vi "Cryotel set mode.vi"() -> ()   [LabVIEW 2019]
panel:
  in  "PWOUT":dbl
  out "Step #":i32
  out "Command sent":string
  in  "milliseconds to wait":u32=1000
  out "read string array 2":string[](array[string])
  in  "Select command set":u16(ring) items=["Satus", "Constant power", "Target temperature", "Cooler OFF ", "Cooler ON", "Set power "]
  out "read string array":string[](array[string])
  in  "VISA Resource (write)":refnum<visa-resource-name>="COM1"
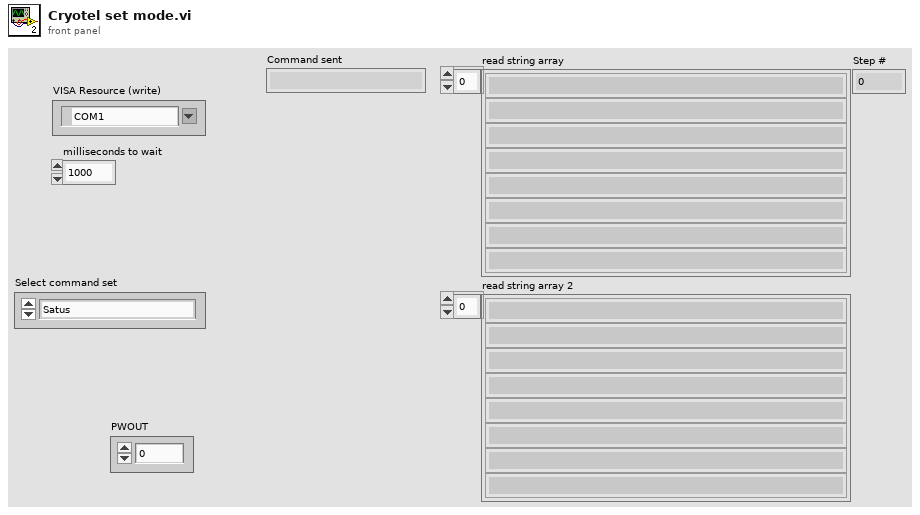
[diagram p1: front panel]
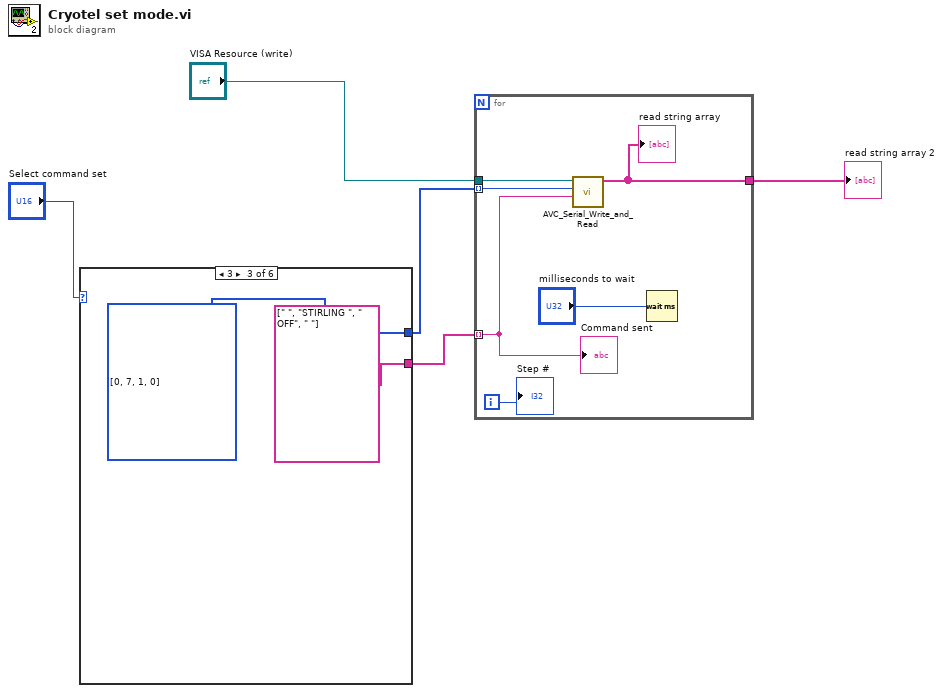
[diagram p0: block diagram]
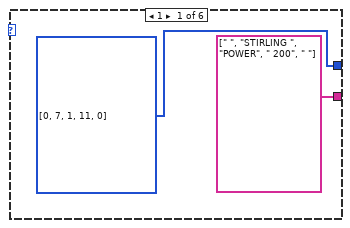
[diagram p2: hidden frame]
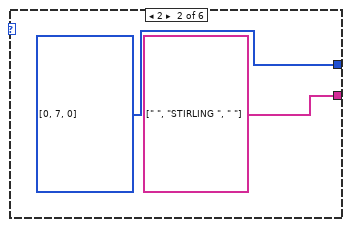
[diagram p3: hidden frame]
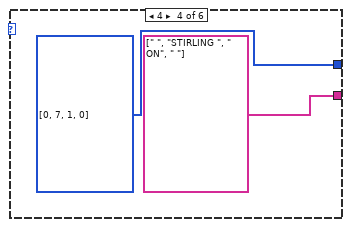
[diagram p4: hidden frame]
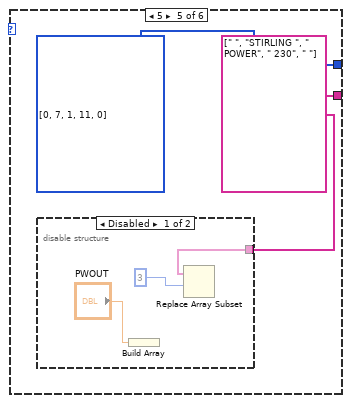
[diagram p5: hidden frame]
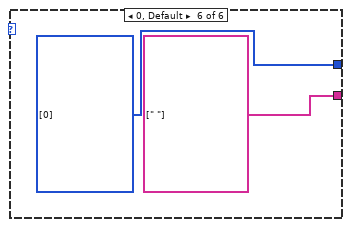
[diagram p7: hidden frame]
diagram:
  n1 = case shown="3" "Select command set" {
    tunnel: [w7 w9 w11 w13 w15 w20] -> w4
    tunnel: [string[] [" ", "STIRLING ", "POWER", " 200", " "] string[] [" ", "STIRLING ", " "] string[] [" ", "STIRLING ", " OFF", " "] string[] [" ", "STIRLING ", " ON", " "] w14 string[] [" "]] -> w3
    frame 1 {
      w7 = u16[] [0, 7, 1, 11, 0] items=["STATUS", "COOLER", "E", "ERROR", "KD", "KI", "KP", "LOGIN", "LOGOUT", "MODE", "P", "PWOUT", "SENSOR", "TC", "TEMP RJ", "TTARGET", "VERSION"]
    }
    frame 2 {
      w9 = u16[] [0, 7, 0] items=["STATUS", "COOLER", "E", "ERROR", "KD", "KI", "KP", "LOGIN", "LOGOUT", "MODE", "P", "PWOUT", "SENSOR", "TC", "TEMP RJ", "TTARGET", "VERSION"]
    }
    frame 3 {
      w11 = u16[] [0, 7, 1, 0] items=["STATUS", "COOLER", "E", "ERROR", "KD", "KI", "KP", "LOGIN", "LOGOUT", "MODE", "P", "PWOUT", "SENSOR", "TC", "TEMP RJ", "TTARGET", "VERSION"]
    }
    frame 4 {
      w13 = u16[] [0, 7, 1, 0] items=["STATUS", "COOLER", "E", "ERROR", "KD", "KI", "KP", "LOGIN", "LOGOUT", "MODE", "P", "PWOUT", "SENSOR", "TC", "TEMP RJ", "TTARGET", "VERSION"]
    }
    frame 5 {
      w14 = string[] [" ", "STIRLING ", " POWER", " 230", " "]
      w15 = u16[] [0, 7, 1, 11, 0] items=["STATUS", "COOLER", "E", "ERROR", "KD", "KI", "KP", "LOGIN", "LOGOUT", "MODE", "P", "PWOUT", "SENSOR", "TC", "TEMP RJ", "TTARGET", "VERSION"]
      n2 = disable-structure shown="Disabled" {
        disable-tunnel: w14 -> [w18 _]
        frame Disabled {
          n3 = Build Array("PWOUT") -> ()  [unwired: 1 out]
          n4 = Replace Array Subset(array=w18, index=3) -> ()  [unwired: 1 in, 1 out]
        }
        frame Enabled {
        }
      }
    }
    frame 0, Default {
      w20 = u16[] [0] items=["STATUS", "COOLER", "E", "ERROR", "KD", "KI", "KP", "LOGIN", "LOGOUT", "MODE", "P", "PWOUT", "SENSOR", "TC", "TEMP RJ", "TTARGET", "VERSION"]
    }
  }
  n5 = for {
    tunnel: "VISA Resource (write)" -> [w26]
    tunnel: w4 -> [w25] mode=indexing
    tunnel: [w24] -> w1
    tunnel: w3 -> [w23] mode=indexing
    i -> [w21]
    n6 = call "AVC_Serial_Write_and_Read.vi"("Command Options"=w23, "Command"=w25, "VISA Resource (write)"=w26) -> ("read string array"=w24:string[])  [unwired: 8 in]
    "read string array" <- w24
    n7 = Wait (ms)(milliseconds to wait="milliseconds to wait") -> ()  [unwired: 1 out]
    "Command sent" <- w23
    "Step #" <- w21
  }
  "read string array 2" <- w1
